vi "Delete Tree.vi"(7 "Tree ID":string, 8 "Error In":errorcluster, 11 "Tree Manager":T1) -> (0 "Error Out":errorcluster, 3 "Tree Manager":T1)   [LabVIEW 2016, in "Tree Manager.lvclass"]
doc: "Delete Tree and all its children. \n\nIf any of the deleted Trees contained attributes of Tree Data.lvclass data type, those attributes will be realeased with the Release.vi dynamically dispatched method.\n\nFor safety purposes this uses not only the specified Tree Data types but all Tree Data types that match from memory."
uses:
  Tree Manager.lvclass
  Typedefs/Session Handle.ctl
  Tree Manager.lvclass/Tree Manager.ctl
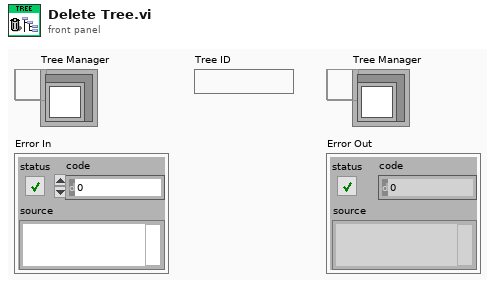
[diagram p1: front panel]
types:
  T1 = typedef "Tree Manager.lvclass/Session Handle.ctl" = refnum<data-value>
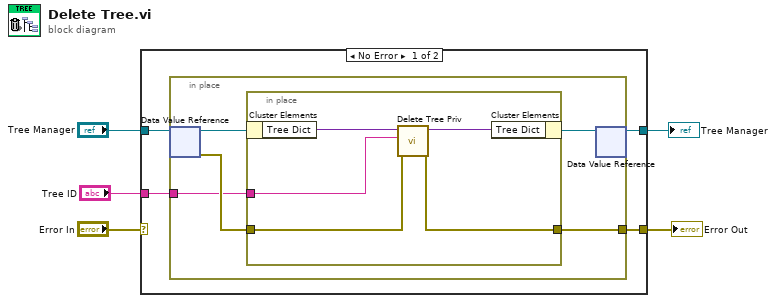
[diagram p0: block diagram]
diagram:
  n1 = case shown="No Error" "Error In" {
    selector: "Error In" -> [_ w20]
    tunnel: "Tree Manager" -> [w9 w21]
    tunnel: [w8 w21] -> w4
    tunnel: [w7 w20] -> w2
    tunnel: "Tree ID" -> [w6 _]
    frame No Error {
      n2 = in-place {
        in-place-border: [w13] -> w7
        in-place-border: w6 -> [w10]
        n3 = in-place-dvr #1(w9) -> (w14:refnum<class "Tree Manager.lvclass">, w11:errorcluster)
        n4 = in-place {
          in-place-border: [w16] -> w13
          in-place-border: w11 -> [w17]
          in-place-border: w10 -> [w15]
          n5 = in-place-cluster #2(w14) -> ("Tree Dict"=w19:variant)
          n6 = call "Delete Tree Priv.vi"("Error In"=w17, "Unique ID"=w15, "Tree Dictionary In"=w19) -> ("Error Out"=w16:errorcluster, "Tree Dictionary Out"=w18:variant)  [unwired: 7 in]
          n7 = in-place-cluster #2("Tree Dict"=w18) -> (w12:refnum<class "Tree Manager.lvclass">)
        }
        n8 = in-place-dvr #1(w12) -> (w8:T1)  [unwired: 1 out]
      }
    }
    frame Error {
    }
  }
  "Tree Manager" <- w4
  "Error Out" <- w2
